vi "cont_update (SubVI).vi"(8 "Array In":i32[](array[numeric]), 10 "name or relative path":string, 11 "Base Path":path) -> (3 "Array Out":i32[](array[numeric]))   [LabVIEW 2013]
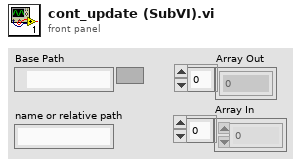
[diagram p1: front panel]
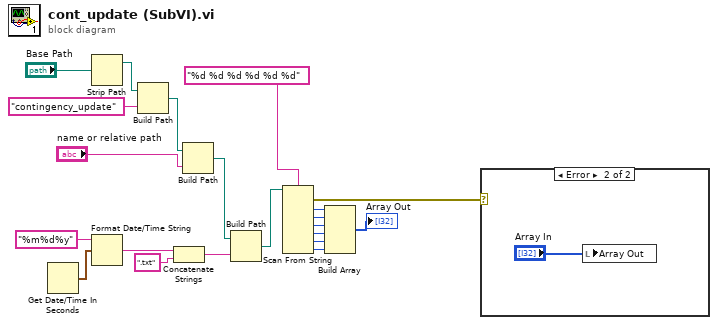
[diagram p0: block diagram]
diagram:
  n1 = Get Date/Time In Seconds() -> (seconds since 1Jan1904=w10:timestamp)
  n2 = Strip Path(path="Base Path") -> (stripped path=w6:path)  [unwired: 1 out]
  n3 = Format Date/Time String(time format string (%c)="%m%d%y", seconds (now)=w10) -> (date/time string=w12:string)  [unwired: 1 in]
  n4 = Build Path(base path=w6, name or relative path="contingency_update") -> (appended path=w8:path)
  n5 = Concatenate Strings(w12, ".txt" ("string")) -> (w14:string)
  n6 = Build Path(base path=w8, name or relative path="name or relative path") -> (appended path=w1:path)
  n7 = Build Path(base path=w1, name or relative path=w14) -> (appended path=w15:path)
  n8 = Scan From String("%d %d %d %d %d %d" ("format string"), w15) -> (w4:errorcluster, output 1=w17:i32, output 2=w18:i32, output 3=w19:i32, output 4=w20:i32, output 5=w3:i32, output 6=w2:i32)  [unwired: 7 in, 1 out]
  n9 = Build Array(w17, w18, w19, w20, w3, w2) -> (→"Array Out":i32[])
  n10 = case shown="Error" w4 {
    frame No Error {
    }
    frame Error {
      n11 = local write "Array Out"("Array In") -> ()
    }
  }
